vi "CRYGet Equal Category.vi"(10 "Current StepName":string, 11 "Find CategoryName":string) -> (2 "setup flattened Array out":T1(array[cluster]), 3 "Find Flag":bool)   [LabVIEW 2013]
uses:
  CRYProject Editor Global.vi
  CRYSystem/Calibration/SubVI/CRYCal Global.vi
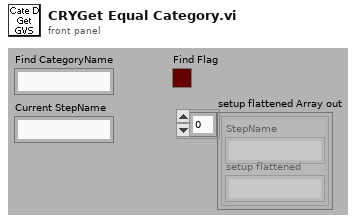
[diagram p1: front panel]
types:
  T1 = cluster{"StepName":string, "setup flattened":string}[]
  T2 = cluster{"StepName":string, "setup flattened":string}
  T3 = typedef "CRYStep.ctl" = cluster{"No.VI":i32, "Category":string, "StepName":string, "Seq setup flattened":string, "Comment":string, "Steps config.":bool[], "Jump config":i32[], "Start":dbl, "Increment":dbl, "Name":string, "Unit":string, "Y data":u16, "Y prefix":string, "Y dB ref":dbl, "Y unit":string, "Repeat State Array":cluster{"Start":dbl, "Increment":dbl, "Count":i32, "Num":i32}[]}
  T4 = typedef "CRYTS.ctl" = cluster{"No.TS":u16, "TS File Path":path, "TS Name":string, "EditStepName":string, "Steps":T3[], "New State":bool, "Change State":bool, "Flattened CurveLib Data":string, "Document Data":string, "EditStepNo":u16, "Operator Start File":string, "Sequence Type":string, "Sequence Language":string}
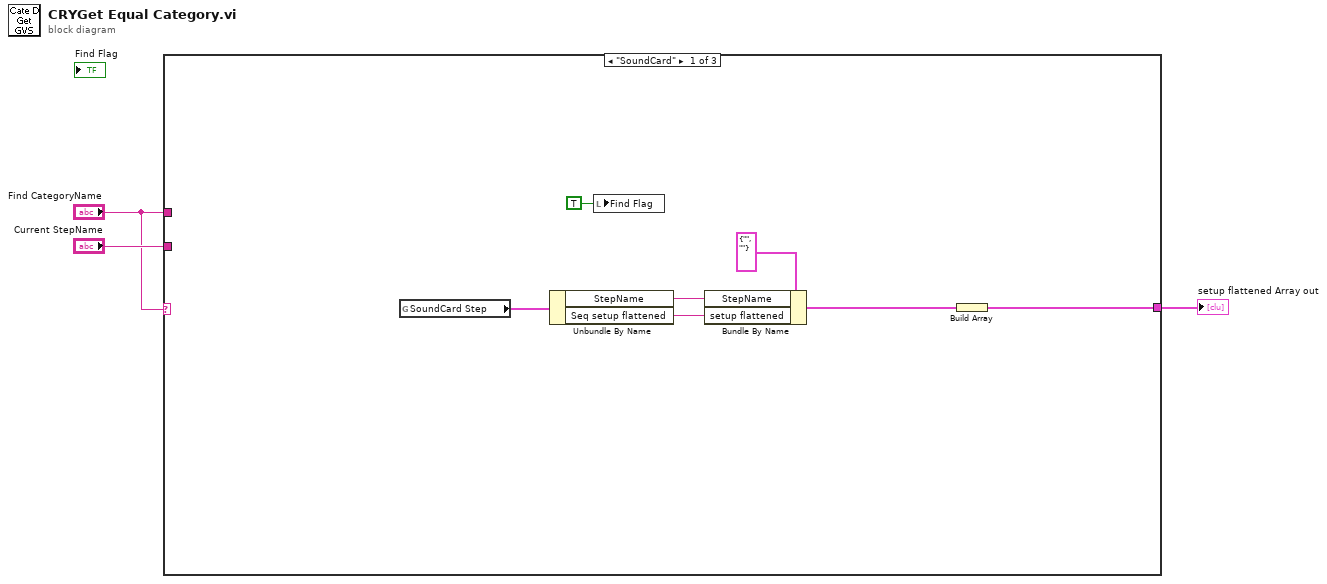
[diagram p0: block diagram]
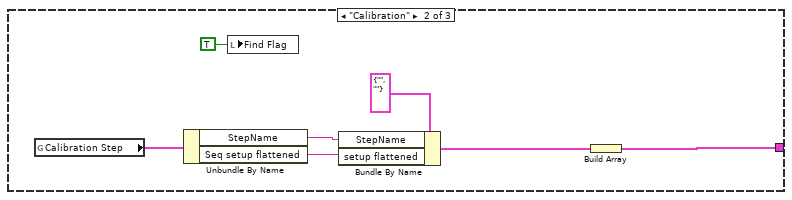
[diagram p2: hidden frame]
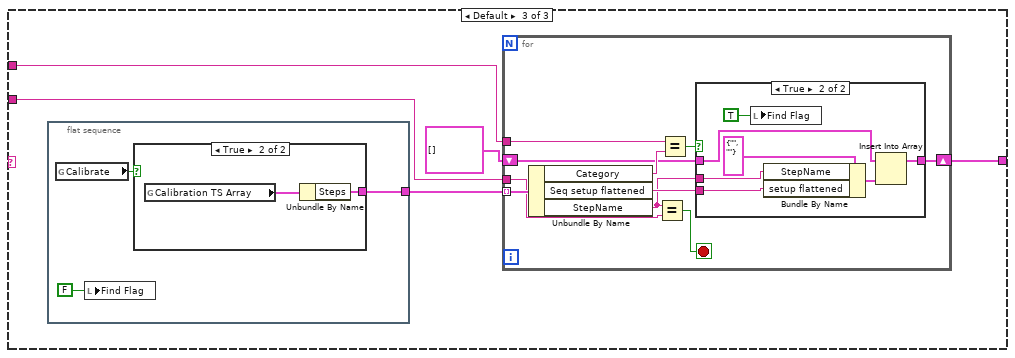
[diagram p3: hidden frame]
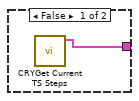
[diagram p4: hidden frame]
diagram:
  n1 = case shown="\"SoundCard\"" "Find CategoryName" {
    tunnel: "Find CategoryName" -> [_ _ w22]
    tunnel: "Current StepName" -> [_ _ w21]
    tunnel: [w4 w11 w19] -> w2
    frame "SoundCard" {
      n2 = global read "CRYProject Editor Global.vi" "SoundCard Step"() -> (w9:T3)
      n3 = Unbundle By Name(w9) -> ("StepName"=w8:string, "Seq setup flattened"=w7:string)
      n4 = local write "Find Flag"(TRUE) -> ()
      n5 = Bundle By Name(cluster=T2 {"StepName"="", "setup flattened"=""} ("output cluster"), "StepName"=w8, "setup flattened"=w7) -> (w5:T2)
      n6 = Build Array(w5) -> (w4:T1)
    }
    frame "Calibration" {
      n7 = global read "CRYProject Editor Global.vi" "Calibration Step"() -> (w16:T3)
      n8 = Unbundle By Name(w16) -> ("StepName"=w15:string, "Seq setup flattened"=w14:string)
      n9 = local write "Find Flag"(TRUE) -> ()
      n10 = Bundle By Name(cluster=T2 {"StepName"="", "setup flattened"=""} ("output cluster"), "StepName"=w15, "setup flattened"=w14) -> (w12:T2)
      n11 = Build Array(w12) -> (w11:T1)
    }
    frame Default {
      n12 = flat-sequence {
        tunnel: [w23] -> w18
        frame #0 {
          n13 = global read "CRYCal Global.vi" "Calibrate"() -> (w24:bool)
          n14 = local write "Find Flag"(FALSE ("Find Flag")) -> ()
          n15 = case shown="True" w24 {
            tunnel: [w26 w27] -> w23
            frame False {
              n16 = call "CRYGet Current TS Steps.vi"() -> ("Steps"=w26:T3[])  [unwired: 7 in, 4 out]
            }
            frame True {
              n17 = global read "CRYProject Editor Global.vi" "Calibration TS Array"() -> (w28:T4)
              n18 = Unbundle By Name(w28) -> ("Steps"=w27:T3[])
            }
          }
        }
      }
      n19 = for {
        tunnel: w22 -> [w38]
        tunnel: w18 -> [w37] mode=indexing
        tunnel: w21 -> [w33]
        shift-right: [w31] -> w19
        shift-left: T1 [] -> [w30]
        stop <- w29 stop-if-true
        n20 = Unbundle By Name(w37) -> ("Category"=w36:string, "Seq setup flattened"=w34:string, "StepName"=w32:string)
        n21 = Equal?(x=w32, y=w33) -> (x = y?=w29:bool)
        n22 = Equal?(x=w38, y=w36) -> (x = y?=w35:bool)
        n23 = case shown="True" w35 {
          tunnel: w34 -> [_ w41]
          tunnel: w32 -> [_ w42]
          tunnel: [w39 w45] -> w31
          tunnel: w30 -> [w39 w44]
          frame False {
          }
          frame True {
            n24 = local write "Find Flag"(TRUE) -> ()
            n25 = Bundle By Name(cluster=T2 {"StepName"="", "setup flattened"=""} ("output cluster"), "StepName"=w42, "setup flattened"=w41) -> (w40:T2)
            n26 = Insert Into Array(array=w44, new element=w40) -> (w45:T1)  [unwired: 1 in]
          }
        }
      }
    }
  }
  "setup flattened Array out" <- w2
